vi "Deposition-handler.vi"(8 "error in (no error)":errorcluster, 11 "Object ref in":T1) -> (0 "error out":errorcluster, 3 "Object ref out":T1)   [LabVIEW 2013, in "SLMControl.lvlib" / "SC-Main.lvclass"]
uses:
  SC-Main.lvclass
  Object-reference.ctl
  Deposition-actions.ctl
  Main-actions.ctl
  Enqueue-modes.ctl
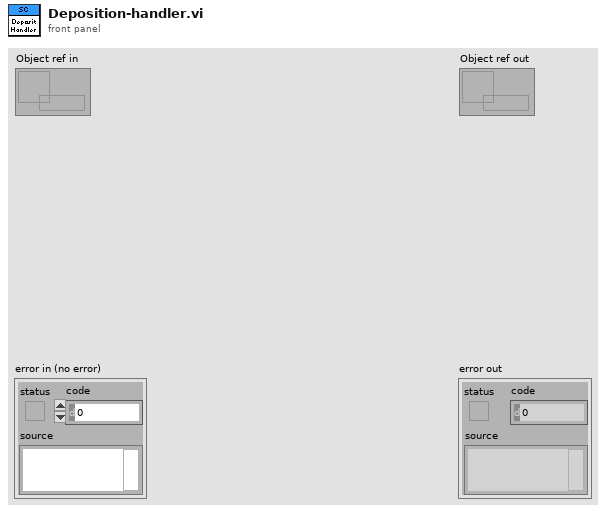
[diagram p1: front panel]
types:
  T1 = typedef "SLMControl.lvlib/SC-Main.lvclass/Object-reference.ctl" = refnum<data-value>
  T2 = typedef "SLMControl.lvlib/SC-Main.lvclass/Deposition-actions.ctl" = enum16{"Idle", "Activate", "Load deposition", "Launch deposition", "Wait for deposition end", "Signal lasing", "Abort", "Reset", "Exit"}
  T3 = typedef "SLMControl.lvlib/SC-Main.lvclass/Enqueue-modes.ctl" = enum16{"Default", "Priority", "Flush"}
  T4 = typedef "SLMControl.lvlib/SC-Main.lvclass/Main-actions.ctl" = enum16{"Idle", "Initialize", "Load configuration", "Save configuration", "Load lasing files", "Load deposition files", "Refresh files", "Clear files", "Open lasing file", "Activate", "Start", "Start deposition cycle", "Start lasing cycle", "Iterate", "Abort", "Stop", "Exit"}
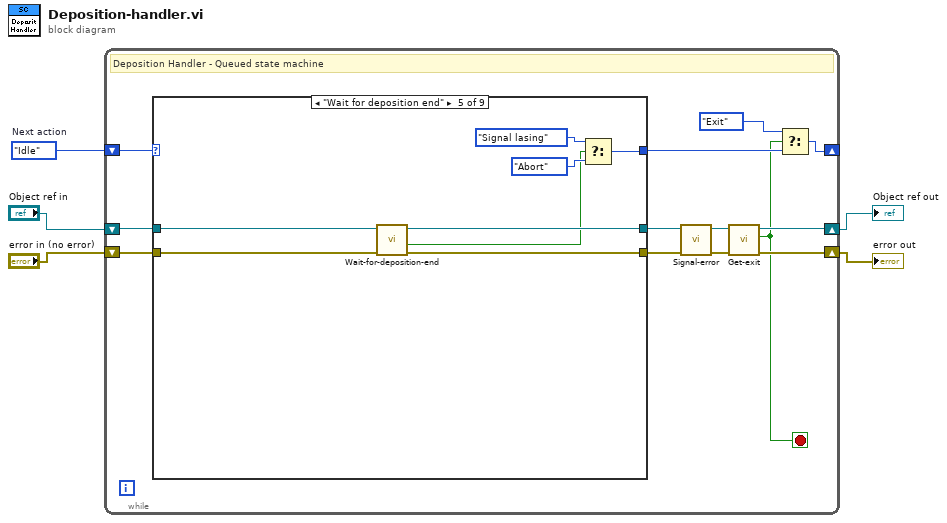
[diagram p0: block diagram]
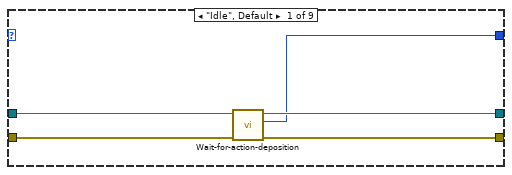
[diagram p2: hidden frame]
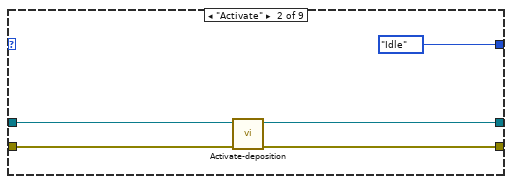
[diagram p3: hidden frame]
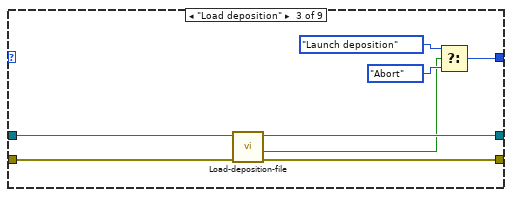
[diagram p4: hidden frame]
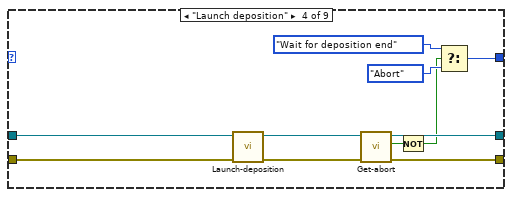
[diagram p5: hidden frame]
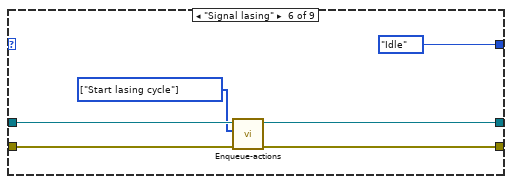
[diagram p6: hidden frame]
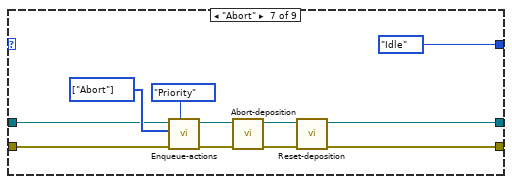
[diagram p7: hidden frame]
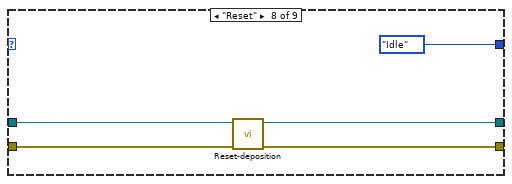
[diagram p8: hidden frame]
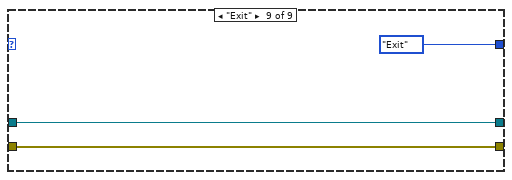
[diagram p9: hidden frame]
diagram:
  w5 = Deposition-actions."Idle"  # Next action
  n1 = while {
    shift-right: [w10] -> _
    shift-left: w5 -> [w18]
    shift-right: [w8] -> w4
    shift-left: "error in (no error)" -> [w17]
    shift-right: [w13] -> w3
    shift-left: "Object ref in" -> [w16]
    stop <- w6 stop-if-true
    # "Deposition Handler - Queued state machine"
    n2 = case shown="\"Wait for deposition end\"" w18 {
      tunnel: w17 -> [w19 w26 w35 w46 w54 w59 w63 w75 w78]
      tunnel: [w21 w24 w30 w38 w49 w58 w68 w73 w78] -> w7
      tunnel: [w20 Deposition-actions."Idle" ("Action Handler states") w34 w43 w53 Deposition-actions."Idle" ("Action Handler states") Deposition-actions."Idle" ("Action Handler states") Deposition-actions."Idle" ("Action Handler states") Deposition-actions."Exit" ("Action Handler states")] -> w11
      tunnel: w16 -> [w23 w27 w36 w47 w55 w60 w64 w76 w79]
      tunnel: [w22 w25 w31 w39 w50 w57 w70 w74 w79] -> w15
      frame "Idle", Default {
        n3 = call "Wait-for-action-deposition.vi"("error in (no error)"=w19, "Object ref in"=w23) -> ("error out"=w21:errorcluster, "Action"=w20:T2, "Object ref out"=w22:T1)  [unwired: 7 in]
      }
      frame "Activate" {
        n4 = call "Activate-deposition.vi"("error in (no error)"=w26, "Object ref in"=w27) -> ("error out"=w24:errorcluster, "Object ref out"=w25:T1)  [unwired: 8 in]
      }
      frame "Load deposition" {
        n5 = call "Load-deposition-file.vi"("error in (no error)"=w35, "Object ref in"=w36) -> ("error out"=w30:errorcluster, "Succes?"=w29:bool, "Object ref out"=w31:T1)  [unwired: 7 in]
        n6 = Select(t=Deposition-actions."Launch deposition" ("Action Handler states"), s=w29, f=Deposition-actions."Abort" ("Action Handler states")) -> (s? t:f=w34:T2)
      }
      frame "Launch deposition" {
        n7 = call "Launch-deposition.vi"("error in (no error)"=w46, "Object ref in"=w47) -> ("error out"=w44:errorcluster, "Object ref out"=w45:T1)  [unwired: 8 in]
        n8 = call "Get-abort.vi"("error in (no error)"=w44, "Object ref in"=w45) -> ("error out"=w38:errorcluster, "Abort"=w40:bool, "Object ref out"=w39:T1)  [unwired: 7 in]
        n9 = Not(x=w40) -> (.not. x?=w37:bool)
        n10 = Select(t=Deposition-actions."Wait for deposition end" ("Action Handler states"), s=w37, f=Deposition-actions."Abort" ("Action Handler states")) -> (s? t:f=w43:T2)
      }
      frame "Wait for deposition end" {
        n11 = call "Wait-for-deposition-end.vi"("error in (no error)"=w54, "Object ref in"=w55) -> ("error out"=w49:errorcluster, "Succes?"=w48:bool, "Object ref out"=w50:T1)  [unwired: 7 in]
        n12 = Select(t=Deposition-actions."Signal lasing" ("Action Handler states"), s=w48, f=Deposition-actions."Abort" ("Action Handler states")) -> (s? t:f=w53:T2)
      }
      frame "Signal lasing" {
        w56 = T4[] [enum."Start lasing cycle"] items=["Idle", "Initialize", "Load configuration", "Save configuration", "Load lasing files", "Load deposition files", "Refresh files", "Clear files", "Open lasing file", "Activate", "Start", "Start deposition cycle", "Start lasing cycle", "Iterate", "Abort", "Stop", "Exit"] ("State array")
        n13 = call "Enqueue-actions.vi"("error in (no error)"=w59, "State array"=w56, "State queue in"=w60) -> ("error out"=w58:errorcluster, "State queue out"=w57:T1)  [unwired: 6 in, 1 out]
      }
      frame "Abort" {
        w66 = T4[] [enum."Abort"] items=["Idle", "Initialize", "Load configuration", "Save configuration", "Load lasing files", "Load deposition files", "Refresh files", "Clear files", "Open lasing file", "Activate", "Start", "Start deposition cycle", "Start lasing cycle", "Iterate", "Abort", "Stop", "Exit"] ("State array")
        n14 = call "Enqueue-actions.vi"("Enqueue mode"=Enqueue-modes."Priority", "error in (no error)"=w63, "State array"=w66, "State queue in"=w64) -> ("error out"=w62:errorcluster, "State queue out"=w65:T1)  [unwired: 5 in, 1 out]
        n15 = call "Abort-deposition.vi"("error in (no error)"=w62, "Object ref in"=w65) -> ("error out"=w69:errorcluster, "Object ref out"=w71:T1)  [unwired: 8 in]
        n16 = call "Reset-deposition.vi"("error in (no error)"=w69, "Object ref in"=w71) -> ("error out"=w68:errorcluster, "Object ref out"=w70:T1)  [unwired: 8 in]
      }
      frame "Reset" {
        n17 = call "Reset-deposition.vi"("error in (no error)"=w75, "Object ref in"=w76) -> ("error out"=w73:errorcluster, "Object ref out"=w74:T1)  [unwired: 8 in]
      }
      frame "Exit" {
      }
    }
    n18 = call "Signal-error.vi"("error in (no error)"=w7, "Data in"=w15) -> ("error out"=w12:errorcluster, "Data out"=w14:T1)  [unwired: 8 in]
    n19 = call "Get-exit.vi"("error in (no error)"=w12, "Object ref in"=w14) -> ("error out"=w8:errorcluster, "Exit?"=w6:bool, "Object ref out"=w13:T1)  [unwired: 7 in]
    n20 = Select(t=Deposition-actions."Exit", s=w6, f=w11) -> (s? t:f=w10:T2)
  }
  "error out" <- w4
  "Object ref out" <- w3
